vi "JYGetCurrentWL.vi"(8 "error in (no error)":errorcluster, 10 "UniqueID":string, 11 "JYMONOLib.IJYMonoReqd In":refnum<k7>) -> (0 "error out":errorcluster, 1 "Units":string, 2 "Current WL":dbl, 3 "JYMONOLib.IJYMonoReqd Out":refnum<k7>)   [LabVIEW 2009]
doc: "JYGetCurrentWL.vi\n\nGets the current wavelength setting of\nthe mono\n\nInputs -\nAutomation Refnum\nUniqueID\nError Cluster\n\n\nOutputs -\nCurrent WL - double; the current wavelength setting\n of the mono\nUnits - string; string description of wavelength units\nError Cluster -"
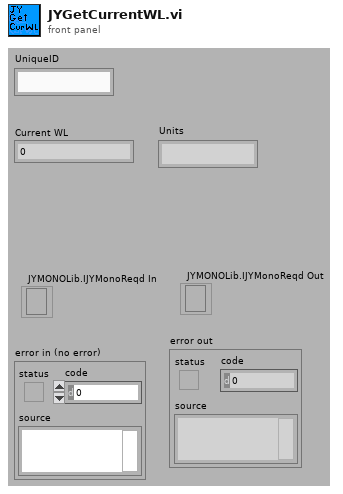
[diagram p1: front panel]
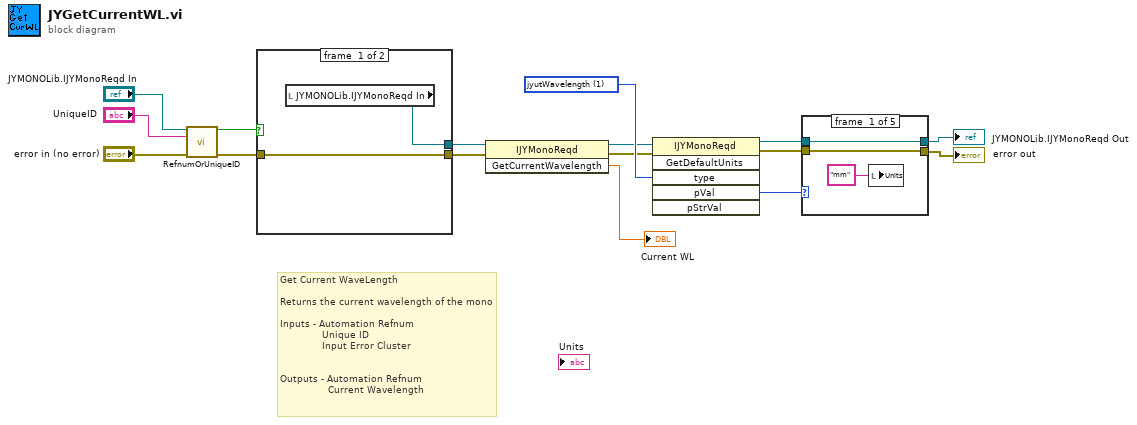
[diagram p0: block diagram]
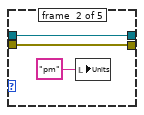
[diagram p2: hidden frame]
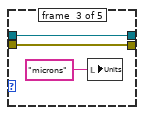
[diagram p3: hidden frame]
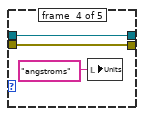
[diagram p4: hidden frame]
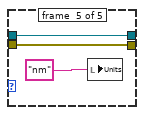
[diagram p5: hidden frame]
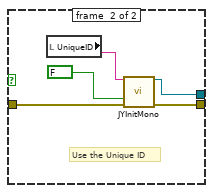
[diagram p6: hidden frame]
diagram:
  w8 = 1 items=["jyutUndefined", "jyutWavelength", "jyutSlitWidth", "jyutTime", "jyutTemperature", "jyutDataUnits", "jyutSpatial", "jyutTotalTypesPlusOne"] ("type")
  # "Get Current WaveLength\n\nReturns the current wavelength of the mono\n\nInputs - Automation Refnum\n              Unique ID\n              Input Error Cluster\n\n\nOutputs - Automation Refnum\n                Current Wavelength"
  n1 = call "RefnumOrUniqueID.vi"("Refnum IN"="JYMONOLib.IJYMonoReqd In", "String in"="UniqueID", "error in (no error)"="error in (no error)") -> ("UseUniqueID"=w12:bool, "error out"=w11:errorcluster)  [unwired: 11 out]
  n2 = case shown="False" w12 {
    tunnel: w11 -> [w18 w21]
    tunnel: [w18 w20] -> w10
    tunnel: [w17 w19] -> w9
    frame #0 {
      n3 = local read "JYMONOLib.IJYMonoReqd In"() -> (w17:refnum<k7>)
    }
    frame #1 {
      # "Use the Unique ID"
      n4 = local read "UniqueID"() -> (w23:string)
      n5 = call "JYInitMono.vi"("Unique ID"=w23, "Force Init"=FALSE, "error in (no error)"=w21) -> ("Mono RefNum out"=w19:refnum<k7>, "error out"=w20:errorcluster)  [unwired: 1 in, 10 out]
    }
  }
  n6 = invoke class="IJYMonoReqd" method="GetCurrentWavelength"(reference=w9, error in=w10) -> (reference out=w7:refnum<k7>, error out=w6:errorcluster, "GetCurrentWavelength"=→"Current WL":dbl)  [unwired: 1 in]
  n7 = invoke class="IJYMonoReqd" method="GetDefaultUnits"(reference=w7, error in=w6, "type"=w8) -> (reference out=w4:refnum<k7>, error out=w2:errorcluster, "pVal"=w5:i32)  [unwired: 3 in, 3 out]
  n8 = case shown="1, Default" w5 {
    tunnel: w4 -> [w25 w28 w31 w34 w37]
    tunnel: [w25 w28 w31 w34 w37] -> w3
    tunnel: w2 -> [w24 w27 w30 w33 w36]
    tunnel: [w24 w27 w30 w33 w36] -> w1
    frame #0 {
      n9 = local write "Units"("mm") -> ()
    }
    frame #1 {
      n10 = local write "Units"("pm") -> ()
    }
    frame #2 {
      n11 = local write "Units"("microns") -> ()
    }
    frame #3 {
      n12 = local write "Units"("angstroms") -> ()
    }
    frame #4 {
      n13 = local write "Units"("nm") -> ()
    }
  }
  "error out" <- w1
  "JYMONOLib.IJYMonoReqd Out" <- w3
